vi "Test App Add Process with Used Name Throws Error.vi"(8 "error in (no error)":errorcluster, 11 "Rig Test in":refnum<class "Application Test.lvclass">) -> (0 "error out":errorcluster, 3 "Rig Test out":refnum<class "Application Test.lvclass">)   [LabVIEW 2020, in "Application Test.lvclass"]
uses:
  Application Test.lvclass
  C:/Program Files (x86)/National Instruments/LabVIEW 2020/vi.lib/Asteme/LUnit/Test Case.lvclass
  Framework/Process/Process.lvclass
  Mock Error Handler/Mock Error Handler.lvclass
  C:/Users/anton/Documents/GitHub/Triarc-Framework/source/Framework/Error Handler Interface/Error Handler Interface.lvclass
  Framework/Process/Process.lvclass/Process.ctl
  Framework/Application/Application.lvclass/Application.ctl
  <vilib>/Asteme/LUnit/Test Case.lvclass/Test Case.ctl
  <vilib>/Asteme/LUnit/LUnit Assertion Result.lvclass/LUnit Assertion Result.ctl
  Framework/Process/Protected/Messaging/Enqueue Message.vi
  Framework/Process/Public/Lifecycle/Get Lifecycle State.vi
  Framework/Application/Private/Add Process to Map.vi
  Framework/Application/Private/Start Idle Processes if Running.vi
  Framework/Process/Protected/SubVIs/Set Context.vi
  <vilib>/Asteme/LUnit/Palette/Fail.vi
  <vilib>/Asteme/LUnit/Palette/Pass.vi
  <vilib>/Asteme/LUnit/Set Assertion Type.vi
  Framework/Process/Protected/Messaging/Request Message.vi
  <vilib>/Asteme/LUnit/Variant to string.vi
  Framework/Process/Private/SubVIs/Wait for finish.vi
  Framework/Process/Private/SubVIs/Set Lifecycle State.vi
  <vilib>/Utility/error.llb/Clear Errors.vi
  Framework/Process/Public/Lifecycle/Leave Process Loop.vi
  <vilib>/Asteme/LUnit/Add test result.vi
  <vilib>/Asteme/LUnit/LUnit Write Passed.vi
  <vilib>/Asteme/LUnit/LUnit Get Test Case.vi
  <vilib>/Asteme/LUnit/Assertion Result/LUnit Get Test Name.vi
  <vilib>/Asteme/LUnit/LUnit Write Message.vi
  <vilib>/Asteme/LUnit/LUnit Write Description.vi
  <vilib>/Asteme/LUnit/LUnit Write Assertion Type.vi
  Framework/Process/Private/SubVIs/Enqueue Request Message.vi
  <vilib>/Asteme/LUnit/Read Test Case Name.vi
  Framework/Application/Application.lvclass
  C:/Users/anton/Documents/GitHub/Triarc-Framework/source/Framework/Process/Process.lvclass
  <vilib>/Utility/error.llb/Error Cluster From Error Code.vi
  Framework/Application/Private/Throw Error If Process Already in App.vi
  Framework/Application/Private/Update Context for Owned Processes.vi
  Framework/Process/Private/SubVIs/Wait for Response Message.vi
  <vilib>/Utility/Data Type/Get Type Information.vi
  <vilib>/Utility/LVClass/Get LV Class Name.vi
  <vilib>/Asteme/LUnit/LUnit Assertion Result.lvclass
  C:/Users/anton/Documents/GitHub/Triarc-Framework/source/Framework/Base/Base.lvclass
  C:/Users/anton/Documents/GitHub/Triarc-Framework/source/Framework/Logging/Logging.lvclass
  C:/Users/anton/Documents/GitHub/Triarc-Framework/source/Framework/Application/Application.lvclass
  C:/Users/anton/Documents/GitHub/Triarc-Framework/source/Framework/Asynchronous Action/Async Action.lvclass
  <vilib>/Asteme/LUnit/Test Case.lvclass
  C:/Users/anton/Documents/GitHub/Triarc-Framework/source/Framework Test/Process Test/Process Test.lvclass
  C:/Users/anton/Documents/GitHub/Triarc-Framework/source/Framework Test/Base Class Test/Base Test.lvclass
  C:/Users/anton/Documents/GitHub/Triarc-Framework/source/Framework Test/Application Test/Application Test.lvclass
  C:/Users/anton/Documents/GitHub/Triarc-Framework/source/Framework Test/Mock Error Handler/Mock Error Handler.lvclass
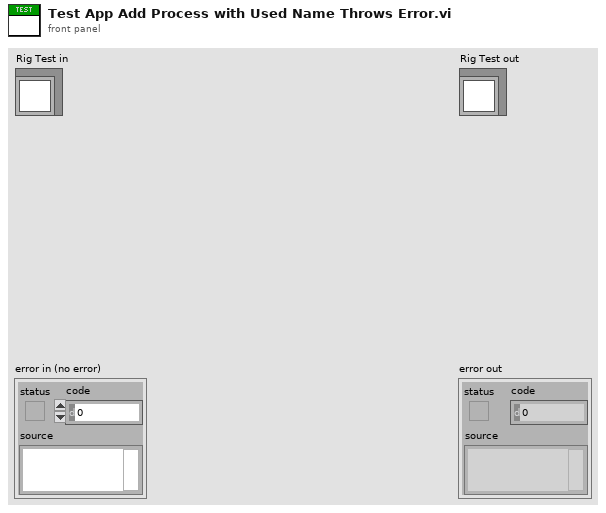
[diagram p1: front panel]
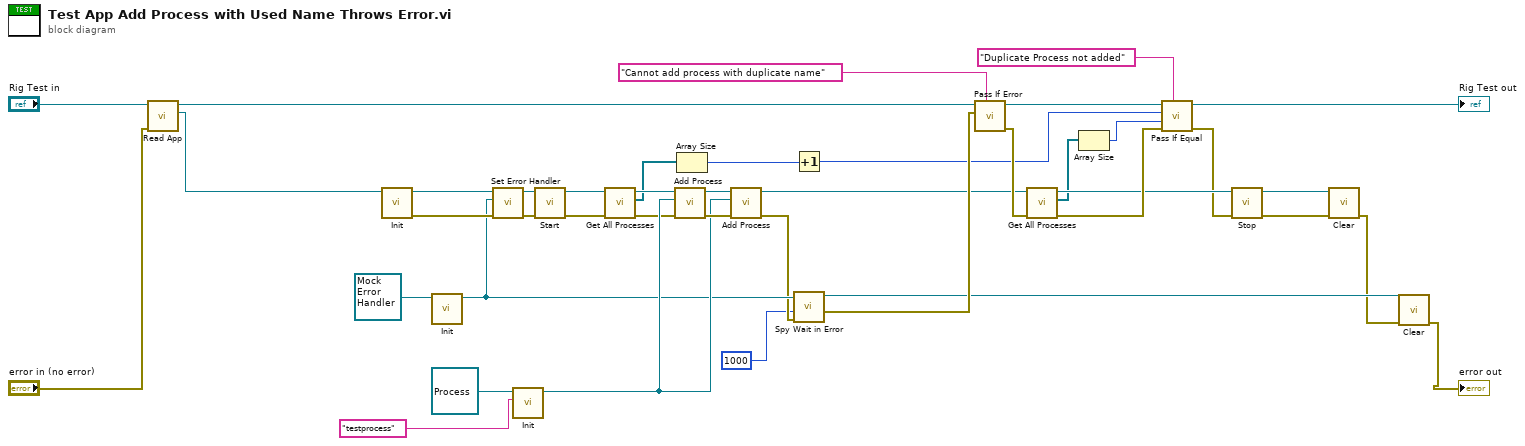
[diagram p0: block diagram]
diagram:
  n1 = call "Read App.vi"("error in (no error)"="error in (no error)", "Application Test In"="Rig Test in") -> ("App out"=w40:refnum<class "Application.lvclass">, "Application Test Out"=w30:refnum<class "Application Test.lvclass">)  [unwired: 7 in, 1 out]
  n2 = call-dynamic "Init.vi"("Process In"=w40) -> ("error out"=w31:errorcluster, "Process Out"=w25:refnum<class "Application.lvclass">)  [unwired: 9 in]
  n3 = call-dynamic "Init.vi"("Mock Error Handler In"=refnum<class "Mock Error Handler.lvclass"> refnum ("Mock Error Handler.lvclass")) -> ("Mock Error Handler Out"=w22:refnum<class "Mock Error Handler.lvclass">)  [unwired: 9 in, 1 out]
  n4 = call "Set Error Handler.vi"("error in (no error)"=w31, "Error Handler"=w22, "Process In"=w25) -> ("error out"=w26:errorcluster, "Process Out"=w24:refnum<class "Application.lvclass">)  [unwired: 7 in]
  n5 = call-dynamic "Init.vi"("Name"="testprocess", "Process In"=refnum<class "Process.lvclass"> refnum ("Process.lvclass")) -> ("Process Out"=w27:refnum<class "Process.lvclass">)  [unwired: 8 in, 1 out]
  n6 = call "Start.vi"("error in (no error)"=w26, "Process In"=w24) -> ("error out"=w32:errorcluster, "Process Out"=w5:refnum<class "Application.lvclass">)  [unwired: 8 in]
  n7 = call "Get All Processes.vi"("error in (no error)"=w32, "Application In"=w5) -> ("error out"=w6:errorcluster, "App Processes"=w3:refnum<class "Process.lvclass">[], "Application Out"=w4:refnum<class "Application.lvclass">)  [unwired: 7 in]
  n8 = call "Add Process.vi"("error in (no error)"=w6, "Process"=w27, "Rig In"=w4) -> ("error out"=w35:errorcluster, "Rig Out"=w38:refnum<class "Application.lvclass">)  [unwired: 7 in]
  n9 = Array Size(array=w3) -> (size(s)=w2:i32)
  n10 = call "Add Process.vi"("error in (no error)"=w35, "Process"=w27, "Rig In"=w38) -> ("error out"=w21:errorcluster, "Rig Out"=w15:refnum<class "Application.lvclass">)  [unwired: 7 in]
  n11 = Increment(x=w2) -> (x+1=w1:i32)
  n12 = call "Spy Wait in Error.vi"("error in (no error)"=w21, "timeout in ms (-1)"=1000, "Mock Error Handler In"=w22) -> ("Errors"=w20:errorcluster, "Mock Error Handler Out"=w19:refnum<class "Mock Error Handler.lvclass">)  [unwired: 4 in, 3 out]
  n13 = call <vilib>:"Pass If Error.vi"("Description"="Cannot add process with duplicate name", "Assert error"=w20, "Test Case In"=w30) -> ("error out"=w34:errorcluster, "Test Case Out"=w12:refnum<class "Application Test.lvclass">)  [unwired: 7 in]
  n14 = call "Get All Processes.vi"("error in (no error)"=w34, "Application In"=w15) -> ("error out"=w16:errorcluster, "App Processes"=w10:refnum<class "Process.lvclass">[], "Application Out"=w14:refnum<class "Application.lvclass">)  [unwired: 7 in]
  n15 = Array Size(array=w10) -> (size(s)=w9:i32)
  n16 = call <vilib>:"Pass If Equal.vi"("Description"="Duplicate Process not added", "error in (no error)"=w16, "Actual"=w9, "Expected"=w1, "Test Case In"=w12) -> ("error out"=w13:errorcluster, "Test Case Out"=→"Rig Test out":refnum<class "Application Test.lvclass">)  [unwired: 5 in]
  n17 = call "Stop.vi"("error in (no error)"=w13, "Process In"=w14) -> ("error out"=w29:errorcluster, "Process Out"=w28:refnum<class "Application.lvclass">)  [unwired: 7 in, 1 out]
  n18 = call-dynamic "Clear.vi"("error in (no error)"=w29, "Application In"=w28) -> ("error out"=w18:errorcluster)  [unwired: 9 in]
  n19 = call-dynamic "Clear.vi"("error in (no error)"=w18, "Mock Process In"=w19) -> ("error out"=→"error out":errorcluster)  [unwired: 9 in]
